vi "Flush Queue.vi"(8 "Error In":errorcluster, 11 "Queue Ref In":refnum<queue>) -> (0 "Error Out":errorcluster, 2 "Remaining Elements":string[](array[string]), 3 "Queue Ref Out":refnum<queue>)   [LabVIEW 2016, in "SLL QSM.lvlib"]
doc: "Removes All Elements from the Queue"
uses:
  SLL QSM.lvlib
  Typedefs/Queue Type.ctl
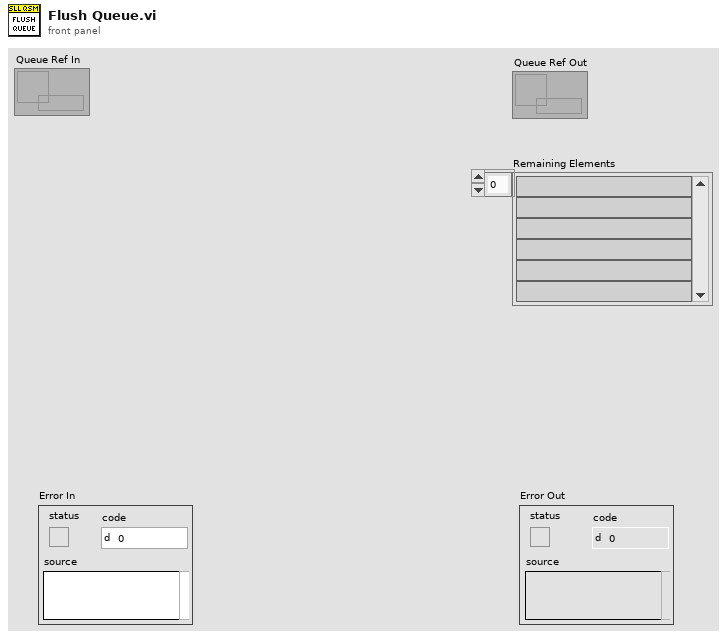
[diagram p1: front panel]
types:
  T1 = typedef "SLL QSM.lvlib/Queue Type.ctl" = cluster{"State":string, "Data":variant}
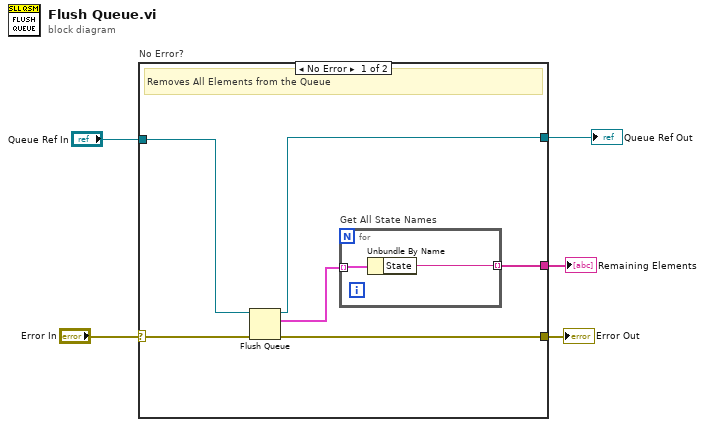
[diagram p0: block diagram]
diagram:
  n1 = case "No Error?" shown="No Error" "Error In" {
    selector: "Error In" -> [w8 w15]
    tunnel: [w11 w15] -> w5
    tunnel: [w9 _] -> w3
    tunnel: "Queue Ref In" -> [w7 w14]
    tunnel: [w6 w14] -> w1
    frame No Error {
      # "Removes All Elements from the Queue"
      n2 = Flush Queue(queue=w7, error in (no error)=w8) -> (queue out=w6:refnum<queue>, remaining elements=w10:T1[], error out=w11:errorcluster)
      n3 = for "Get All State Names" {
        tunnel: w10 -> [w13] mode=indexing
        tunnel: [w12] -> w9 mode=indexing
        n4 = Unbundle By Name(w13) -> ("State"=w12:string)
      }
    }
    frame Error {
    }
  }
  "Error Out" <- w5
  "Remaining Elements" <- w3
  "Queue Ref Out" <- w1
